vi "Path_PPL Folder.vi"() -> (2 "Path Length":i32, 3 "Data Folder Path":path)   [LabVIEW 2019, in "ClassLoader.lvlib"]
doc: "Returns path to the PPL folder. PPLs are assumed to be in a single folder next to each other.\nIf not called from a PPL the VI uses the development/debug path constant \"C:\\Current projects\\WS\\PPL\"."
uses:
  ClassLoader.lvlib
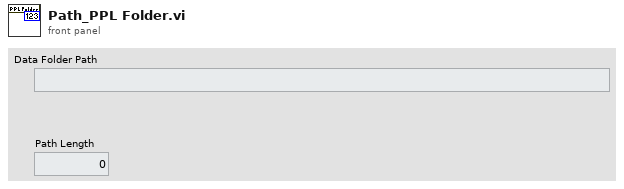
[diagram p1: front panel]
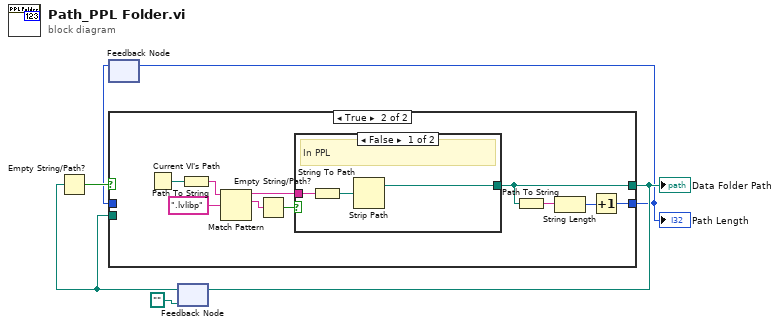
[diagram p0: block diagram]
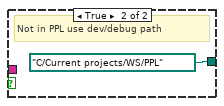
[diagram p3: hidden frame]
diagram:
  n1 = feedback #1() -> (w1:i32)  [unwired: 1 in]
  n2 = feedback #2(path "") -> (w2:path)
  n3 = Empty String/Path?(string/path=w2) -> (empty?=w3:bool)
  n4 = case shown="True" w3 {
    tunnel: [w8 w10] -> w6
    tunnel: w2 -> [w8 _]
    tunnel: [w7 w9] -> w5
    tunnel: w1 -> [w7 _]
    frame False {
    }
    frame True {
      n5 = Current VI's Path() -> (path=w18:path)
      n6 = Path To String(path=w18) -> (string=w17:string)
      n7 = Match Pattern(string=w17, regular expression=".lvlibp") -> (before substring=w15:string, match substring=w14:string)  [unwired: 1 in, 2 out]
      n8 = Empty String/Path?(string/path=w14) -> (empty?=w13:bool)
      n9 = case shown="False" w13 {
        tunnel: [w21 path "C:/Current projects/WS/PPL" ("path")] -> w10
        tunnel: w15 -> [w20 _]
        frame False {
          # "In PPL"
          n10 = String To Path(string=w20) -> (path=w19:path)
          n11 = Strip Path(path=w19) -> (stripped path=w21:path)  [unwired: 1 out]
        }
        frame True {
          # "Not in PPL use dev/debug path"
        }
      }
      n12 = Path To String(path=w10) -> (string=w12:string)
      n13 = String Length(string=w12) -> (length=w11:i32)
      n14 = Increment(x=w11) -> (x+1=w9:i32)
    }
  }
  "Data Folder Path" <- w6
  "Path Length" <- w5
  n15 = feedback-in #1(w5) -> ()
  n16 = feedback-in #2(w6) -> ()
